vi "IntegerTimeToLabTime.vi"(10 "inputTime(msec)":i64) -> (2 "outputTime(mm-ss-sss)":string)   [LabVIEW 2020]
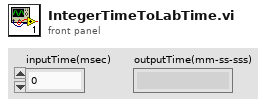
[diagram p1: front panel]
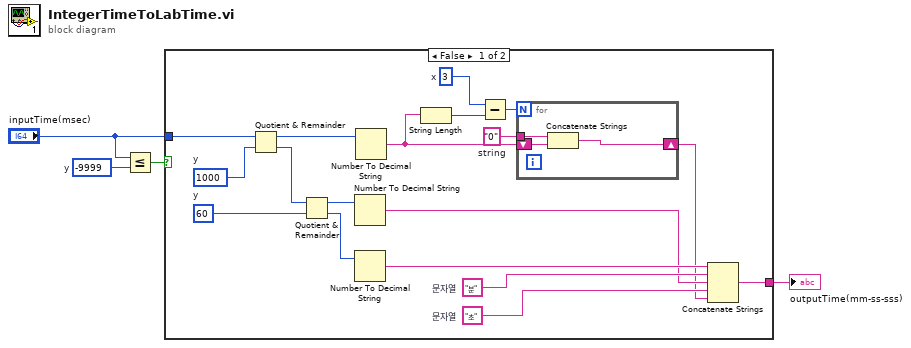
[diagram p0: block diagram]
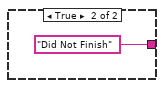
[diagram p2: hidden frame]
diagram:
  w2 = i64 -9999  # y
  n1 = Less Or Equal?(x="inputTime(msec)", y=w2) -> (x <= y?=w1:bool)
  n2 = case shown="False" w1 {
    tunnel: [w21 "Did Not Finish"] -> w4
    tunnel: "inputTime(msec)" -> [w5 _]
    frame False {
      w9 = "0"  # string
      w11 = 3  # x
      w13 = i64 60  # y
      w14 = "초"  # 문자열
      w16 = "분"  # 문자열
      w22 = i64 1000  # y
      n3 = Quotient & Remainder(x=w5, y=w22) -> (x-y*floor(x/y)=w8:i64, floor(x/y)=w20:i64)
      n4 = Quotient & Remainder(x=w20, y=w13) -> (x-y*floor(x/y)=w19:i64, floor(x/y)=w18:i64)
      n5 = Number To Decimal String(number=w19) -> (decimal integer string=w15:string)  [unwired: 1 in]
      n6 = Number To Decimal String ("숫자를 10진수 문자열로")(number=w18) -> (decimal integer string=w17:string)  [unwired: 1 in]
      n7 = Number To Decimal String(number=w8) -> (decimal integer string=w7:string)  [unwired: 1 in]
      n8 = String Length(string=w7) -> (length=w12:i32)
      n9 = Subtract(x=w11, y=w12) -> (x-y=w10:i32)
      n10 = for {
        N: w10 -> [_]
        shift-right: [w24] -> w6
        shift-left: w7 -> [w25]
        tunnel: w9 -> [w23]
        n11 = Concatenate Strings "Concatenate Strings"(w23, w25) -> (w24:string)
      }
      n12 = Concatenate Strings "Concatenate Strings"(w17, w16, w15, w14, w6) -> (w21:string)
    }
    frame True {
    }
  }
  "outputTime(mm-ss-sss)" <- w4
